vi "Get Channel Name.vi"(9 "Channel Name":string, 10 "Channel Path":string, 11 "Root":refnum<k24>) -> (3 "Name":string)   [LabVIEW 2020, in "Workspace MultiY Graph.lvlib"]
uses:
  Workspace MultiY Graph.lvlib
  NationalInstruments.VeriStand.SystemStorage
  NationalInstruments.VeriStand
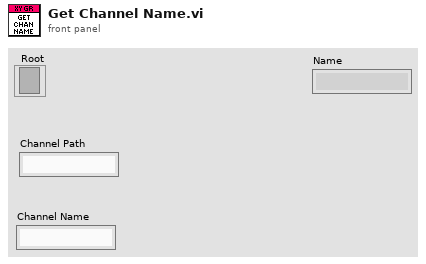
[diagram p1: front panel]
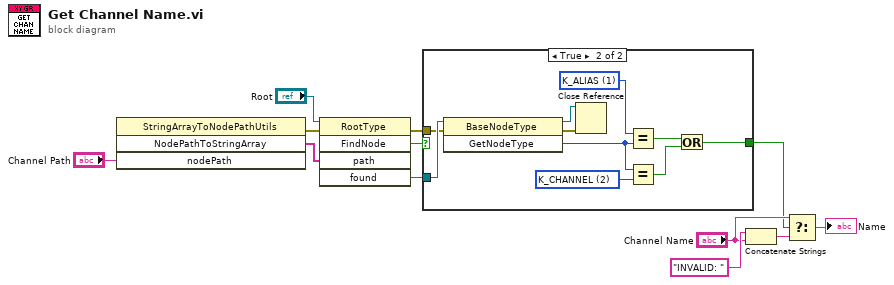
[diagram p0: block diagram]
diagram:
  n1 = invoke class="StringArrayToNodePathUtils" method="NodePathToStringArray"("nodePath"="Channel Path") -> (error out=w11:errorcluster, "NodePathToStringArray"=w10:string[])  [unwired: 3 in, 2 out]
  n2 = invoke class="RootType" method="FindNode"(reference="Root", error in=w11, "path"=w10) -> (error out=w7:errorcluster, "FindNode"=w9:bool, "found"=w8:refnum<k24>)  [unwired: 2 in, 2 out]
  n3 = case shown="True" w9 {
    selector: w9 -> [w13 _]
    tunnel: w8 -> [_ w23]
    tunnel: [w13 w14] -> w3
    tunnel: w7 -> [_ w21]
    frame False {
    }
    frame True {
      w18 = 1 items=["K_BASE", "K_ALIAS", "K_CHANNEL", "K_SECTION", "K_TARGET", "K_TARGETSECTION", "K_ROOT", "K_WAVEFORM"] ("GetNodeType")
      w22 = 2 items=["K_BASE", "K_ALIAS", "K_CHANNEL", "K_SECTION", "K_TARGET", "K_TARGETSECTION", "K_ROOT", "K_WAVEFORM"] ("GetNodeType")
      n4 = invoke class="BaseNodeType" method="GetNodeType"(reference=w23, error in=w21) -> (reference out=w19:refnum<k24>, error out=w20:errorcluster, "GetNodeType"=w17:i32)  [unwired: 1 in]
      n5 = Close Reference(reference=w19, error in (no error)=w20) -> ()  [unwired: 1 out]
      n6 = Equal?(x=w18, y=w17) -> (x = y?=w16:bool)
      n7 = Equal?(x=w17, y=w22) -> (x = y?=w15:bool)
      n8 = Or(x=w16, y=w15) -> (x .or. y?=w14:bool)
    }
  }
  n9 = Concatenate Strings("INVALID: " ("f"), "Channel Name") -> (w1:string)
  n10 = Select(t="Channel Name", s=w3, f=w1) -> (s? t:f=→"Name":string)
